vi "Req_conversion.vi"(5 "Static values in":T4, 7 "error_in":errorcluster, 9 "reqs_bool":T2, 10 "Requirements":T3) -> (0 "error_out":errorcluster, 3 "Reqs_cluster":T1)   [LabVIEW 2017]
uses:
  CONTROLS/Static_values.ctl
  CONTROLS/Requirements.ctl
  CONTROLS/Requirements_boolean.ctl
  CONTROLS/Reqs_cluster.ctl
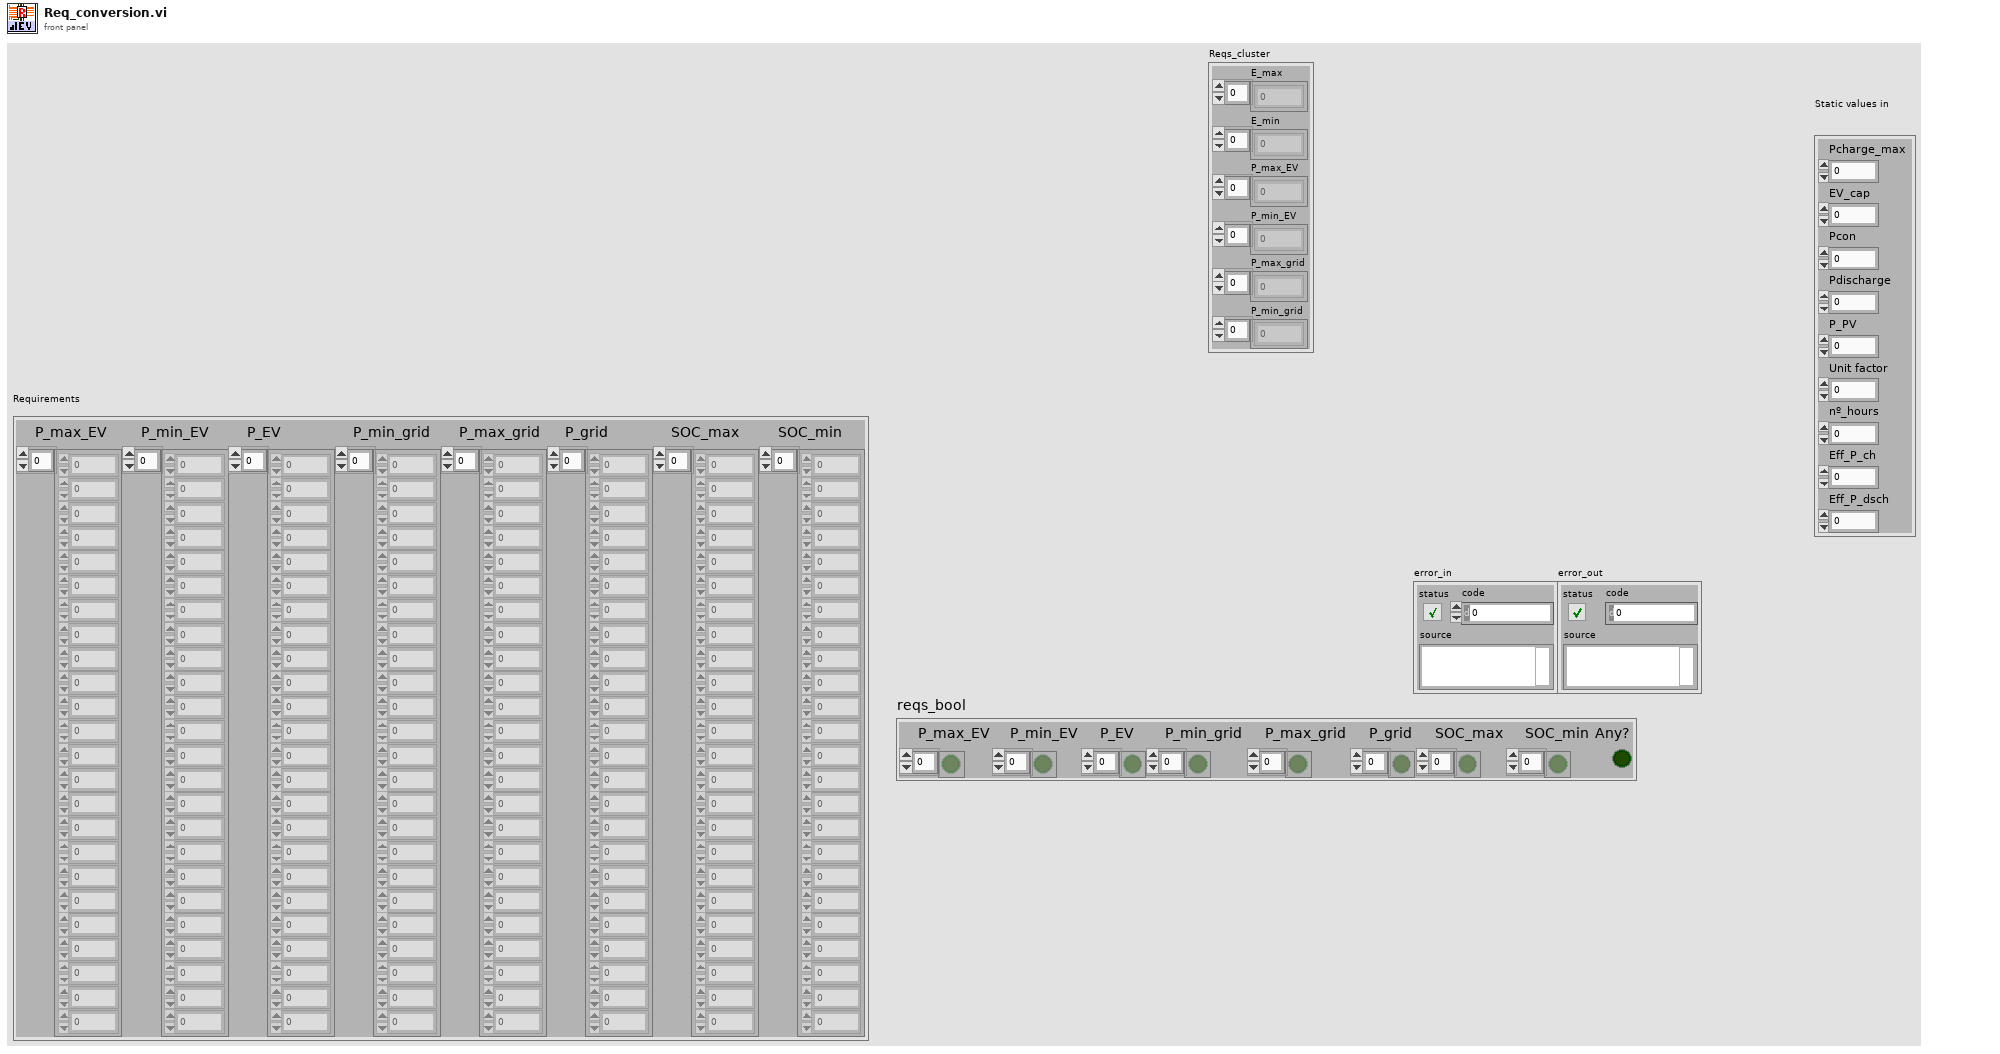
[diagram p1: front panel]
types:
  T1 = typedef "Reqs_cluster.ctl" = cluster{"E_max":dbl[], "E_min":dbl[], "P_max_EV":dbl[], "P_min_EV":dbl[], "P_max_grid":dbl[], "P_min_grid":dbl[]}
  T2 = typedef "Requirements_boolean.ctl" = cluster{"P_max_EV":bool[], "P_min_EV":bool[], "P_EV":bool[], "P_min_grid":bool[], "P_max_grid":bool[], "P_grid":bool[], "SOC_max":bool[], "SOC_min":bool[], "Any?":bool}
  T3 = typedef "Requirements.ctl" = cluster{"P_max_EV":dbl[], "P_min_EV":dbl[], "P_EV":dbl[], "P_min_grid":dbl[], "P_max_grid":dbl[], "P_grid":dbl[], "SOC_max":dbl[], "SOC_min":dbl[]}
  T4 = typedef "Static_values.ctl" = cluster{"Pcharge_max":dbl, "EV_cap":dbl, "Pcon":dbl, "Pdischarge":dbl, "P_PV":dbl, "Unit factor":dbl, "nº_hours":dbl, "Eff_P_ch":dbl, "Eff_P_dsch":dbl}
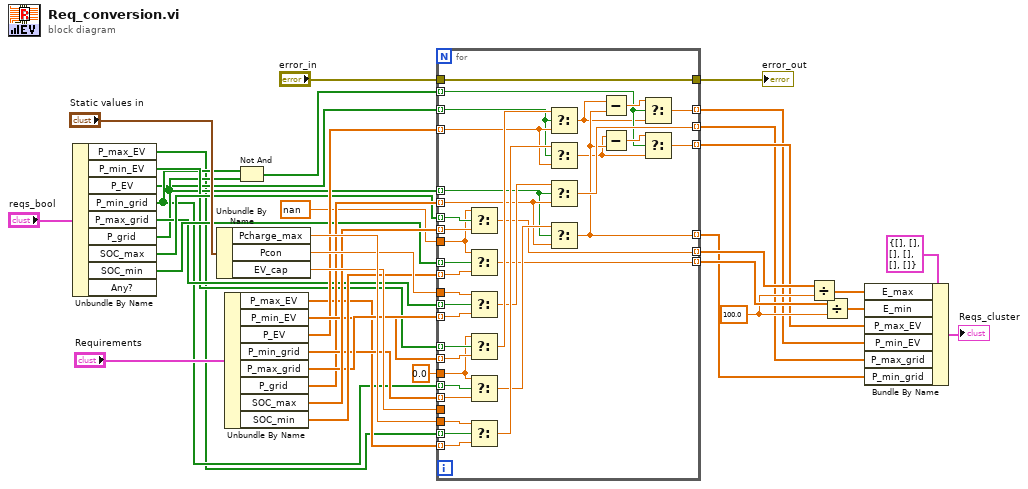
[diagram p0: block diagram]
diagram:
  w32 = 100.0 ("x")
  n1 = Unbundle By Name("reqs_bool") -> ("P_max_EV"=w11:bool[], "P_min_EV"=w15:bool[], "P_EV"=w12:bool[], "P_min_grid"=w13:bool[], "P_max_grid"=w16:bool[], "P_grid"=w14:bool[], "SOC_max"=w18:bool[], "SOC_min"=w17:bool[])  [unwired: 1 out]
  n2 = Unbundle By Name("Static values in") -> ("Pcharge_max"=w34:dbl, "Pcon"=w33:dbl, "EV_cap"=w31:dbl)
  n3 = Unbundle By Name("Requirements") -> ("P_max_EV"=w20:dbl[], "P_min_EV"=w24:dbl[], "P_EV"=w22:dbl[], "P_min_grid"=w23:dbl[], "P_max_grid"=w25:dbl[], "P_grid"=w21:dbl[], "SOC_max"=w27:dbl[], "SOC_min"=w26:dbl[])
  n4 = Not And(1:w14, 2:w13) -> (0:w35:bool[])
  n5 = for {
    tunnel: w11 -> [w47] mode=indexing
    tunnel: w20 -> [w74] mode=indexing
    tunnel: w34 -> [w70]
    tunnel: w15 -> [w44] mode=indexing
    tunnel: w24 -> [w42] mode=indexing
    tunnel: [w62] -> w6 mode=indexing
    tunnel: [w57] -> w7 mode=indexing
    tunnel: w22 -> [w71] mode=indexing
    tunnel: w12 -> [w41] mode=indexing
    tunnel: w16 -> [w48] mode=indexing
    tunnel: w25 -> [w69] mode=indexing
    tunnel: w33 -> [w68]
    tunnel: [w65] -> w5 mode=indexing
    tunnel: w23 -> [w67] mode=indexing
    tunnel: w13 -> [w49] mode=indexing
    tunnel: [w61] -> w4 mode=indexing
    tunnel: w21 -> [w63] mode=indexing
    tunnel: w14 -> [w45] mode=indexing
    tunnel: w35 -> [w56] mode=indexing
    tunnel: w26 -> [w54] mode=indexing
    tunnel: [w53] -> w36 mode=indexing
    tunnel: w17 -> [w55] mode=indexing
    tunnel: w18 -> [w51] mode=indexing
    tunnel: w27 -> [w52] mode=indexing
    tunnel: [w50] -> w37 mode=indexing
    tunnel: w31 -> [_]
    tunnel: [w43] -> w30
    tunnel: "error_in" -> [w43]
    tunnel: nan ("t") -> [w40]
    tunnel: 0.0 ("t") -> [w39]
    n6 = Select(t=w40, s=w51, f=w52) -> (s? t:f=w50:dbl)
    n7 = Select(t=w40, s=w55, f=w54) -> (s? t:f=w53:dbl)
    n8 = Select(t=w68, s=w48, f=w69) -> (s? t:f=w66:dbl)
    n9 = Select(t=w39, s=w44, f=w42) -> (s? t:f=w73:dbl)
    n10 = Select(t=w39, s=w49, f=w67) -> (s? t:f=w64:dbl)
    n11 = Select(t=w70, s=w47, f=w74) -> (s? t:f=w72:dbl)
    n12 = Select(t=w73, s=w41, f=w71) -> (s? t:f=w46:dbl)
    n13 = Select(t=w72, s=w41, f=w71) -> (s? t:f=w58:dbl)
    n14 = Select(t=w66, s=w45, f=w63) -> (s? t:f=w65:dbl)
    n15 = Select(t=w64, s=w45, f=w63) -> (s? t:f=w61:dbl)
    n16 = Subtract(x=w46, y=w61) -> (x-y=w60:dbl)
    n17 = Subtract(x=w58, y=w61) -> (x-y=w59:dbl)
    n18 = Select(t=w60, s=w56, f=w46) -> (s? t:f=w62:dbl)
    n19 = Select(t=w59, s=w56, f=w58) -> (s? t:f=w57:dbl)
  }
  "error_out" <- w30
  n20 = Divide(x=w37, y=w32) -> (x/y=w9:dbl[])
  n21 = Divide(x=w36, y=w32) -> (x/y=w8:dbl[])
  n22 = Bundle By Name(cluster=T1 {"E_max"=[], "E_min"=[], "P_max_EV"=[], "P_min_EV"=[], "P_max_grid"=[], "P_min_grid"=[]}, "E_max"=w9, "E_min"=w8, "P_max_EV"=w7, "P_min_EV"=w6, "P_max_grid"=w5, "P_min_grid"=w4) -> (→"Reqs_cluster":T1)
